vi "ConnectCore.vi"(8 "error in (no error)":errorcluster, 9 "Fully Qualified Name":string, 10 "Connection String":string, 11 "GRPCClient in":refnum<class "MicronGRPCClient.lvclass">) -> (0 "error out":errorcluster, 3 "GRPCClient out":refnum<class "MicronGRPCClient.lvclass">)   [LabVIEW 2019, in "MicronGRPCClient.lvclass"]
uses:
  MicronGRPCClient.lvclass
  MicronGRPCClient.lvclass/MicronGRPCClient.ctl
  <vilib>/SLL Toolkit/SLL String/_SubVIs/String to 1D String Array.vi
  Generated/MicronGRPCGeneratedClient/MicronGRPCGeneratedClient.lvlib
  <vilib>/SLL Toolkit/SLL String/SLL String.lvlib
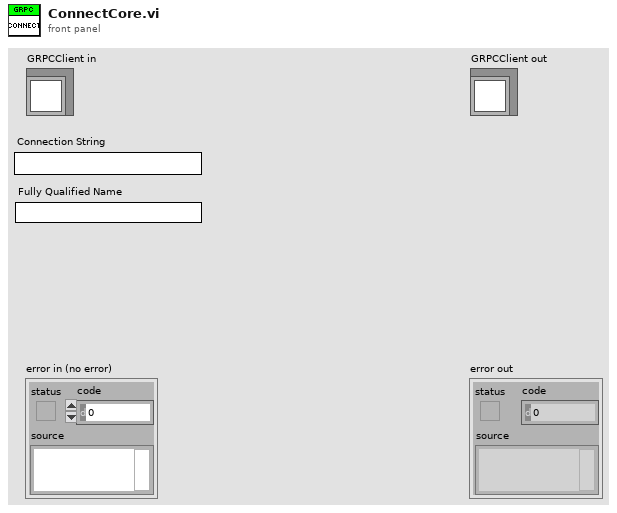
[diagram p1: front panel]
types:
  T1 = typedef "MicronGRPCClient.lvclass/InternalCluster.ctl" = cluster{"ServiceDetails":T2, "gRPCDetails":T3}
  T2 = typedef "MicronClient.lvclass/ServiceDetails.ctl" = cluster{"MicronPath":path, "Network":string, "ServiceID":string, "Port":i32, "FullyQualifiedName":string, "UI":string, "Args":string, "Mode":string, "AutoRestartOnError?":bool, "Simulate?":bool}
  T3 = typedef "gRPCDetails.ctl" = cluster{"ConnectionString":string, "ID":T4, "PackageName":string, "ServiceName":string}
  T4 = typedef "grpc-lvsupport-release.lvlib/grpcId.ctl" = u64
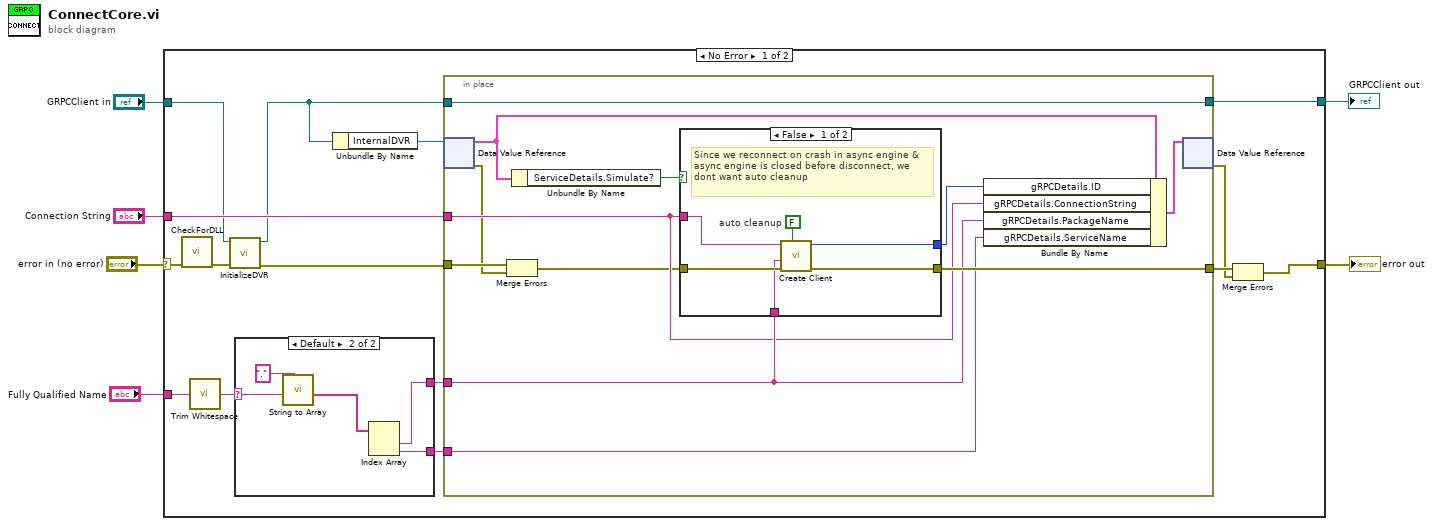
[diagram p0: block diagram]
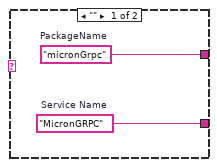
[diagram p3: hidden frame]
diagram:
  n1 = case shown="No Error" "error in (no error)" {
    selector: "error in (no error)" -> [w15 w48]
    tunnel: "Connection String" -> [w14 _]
    tunnel: [w21 w49] -> w5
    tunnel: [w12 w48] -> w3
    tunnel: "Fully Qualified Name" -> [w19 _]
    tunnel: "GRPCClient in" -> [w8 w49]
    frame No Error {
      n2 = call "CheckForDLL.vi"("error in"=w15) -> ("error out"=w10:errorcluster)  [unwired: 10 in]
      n3 = call <vilib>:"Trim Whitespace.vi"("string"=w19) -> ("trimmed string"=w18:string)  [unwired: 1 in]
      n4 = call "InitializeDVR.vi"("error in (no error)"=w10, "MicronGRPCClient in"=w8) -> ("error out"=w9:errorcluster, "MicronGRPCClient out"=w7:refnum<class "MicronGRPCClient.lvclass">)  [unwired: 8 in]
      n5 = case shown="Default" w18 {
        selector: w18 -> [_ w47]
        tunnel: [w42 w44] -> w16
        tunnel: [w41 w43] -> w17
        frame "" {
          w41 = "MicronGRPC"  # Service Name
          w42 = "micronGrpc"  # PackageName
        }
        frame Default {
          n6 = call-poly <vilib>:"String to Array.vi"("Delimiter (,)"=".", "String"=w47) -> ("Array[]"=w45:string[])  [unwired: 6 in]
          n7 = Index Array(array=w45) -> (element #1=w44:string, element #2=w43:string)  [unwired: 2 in]
        }
      }
      n8 = Unbundle By Name(w7) -> ("InternalDVR"=w13:refnum<data-value>)
      n9 = in-place {
        in-place-border: [w24] -> w21
        in-place-border: [w32] -> w20
        in-place-border: w17 -> [w31]
        in-place-border: w16 -> [w30]
        in-place-border: w7 -> [w24]
        in-place-border: w9 -> [w28]
        in-place-border: w14 -> [w27]
        n10 = in-place-dvr #1(w13) -> (w26:T1, w22:errorcluster)
        n11 = Merge Errors(w28, w22) -> (w23:errorcluster)
        n12 = Unbundle By Name(w26) -> ("ServiceDetails.Simulate?"=w29:bool)
        n13 = case shown="False" w29 {
          tunnel: w27 -> [w39 _]
          tunnel: [w38 _] -> w33
          tunnel: w23 -> [w37 w40]
          tunnel: [w36 w40] -> w32
          tunnel: w30 -> [w35 _]
          frame False {
            w34 = FALSE  # auto cleanup
            # "Since we reconnect on crash in async engine & async engine is closed before disconnect, we dont want auto cleanup"
            n14 = call "Create Client.vi"("auto cleanup"=w34, "error in"=w37, "package"=w35, "address"=w39) -> ("error out"=w36:errorcluster, "gRPC ID Out"=w38:T4)  [unwired: 6 in]
          }
          frame True {
          }
        }
        n15 = Bundle By Name(cluster=w26, "gRPCDetails.ID"=w33, "gRPCDetails.ConnectionString"=w27, "gRPCDetails.PackageName"=w30, "gRPCDetails.ServiceName"=w31) -> (w25:T1)
        n16 = in-place-dvr #1(w25) -> (w11:errorcluster)  [unwired: 1 out]
      }
      n17 = Merge Errors(w20, w11) -> (w12:errorcluster)
    }
    frame Error {
    }
  }
  "error out" <- w3
  "GRPCClient out" <- w5
